vi "Verify as JSON.vi"(7 "Test VI (caller)":string, 8 "error in":errorcluster, 10 "Anything":variant, 11 "TestCase":refnum<class "TestCase.lvclass">) -> (0 "error out":errorcluster, 3 "TestCase":refnum<class "TestCase.lvclass">)   [LabVIEW 2020, in "VITester.Extension.lvlib"]
uses:
  VITester.Extension.lvlib
  <vilib>/addons/_JKI Toolkits/VI Tester/TestCase.llb/TestCase.lvclass
  Approval Tests/Approval Tests.lvlib
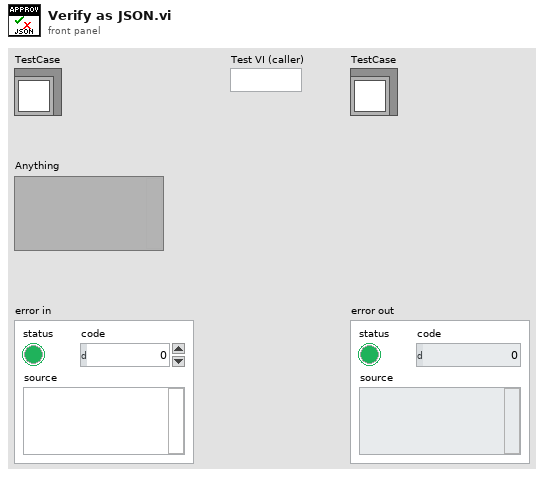
[diagram p1: front panel]
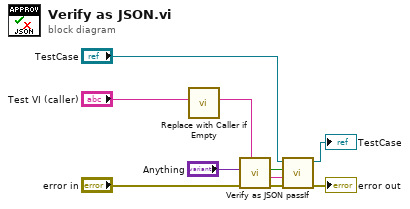
[diagram p0: block diagram]
diagram:
  n1 = call "Replace with Caller if Empty.vi"("Test VI (caller) in"="Test VI (caller)") -> ("Test VI (caller) out"=w2:string)  [unwired: 10 in]
  n2 = call "Verify as JSON.vi"("Test VI (caller)"=w2, "error in"="error in", "Anything"="Anything") -> ("error out"=w9:errorcluster, "Failure Message"=w4:string, "Passed?"=w5:bool)  [unwired: 6 in]
  n3 = call-dynamic "passIf.vi"("error in (no error)"=w9, "message (\"\")"=w4, "pass"=w5, "TestCase in"="TestCase") -> ("error out"=→"error out":errorcluster, "TestCase out"=→"TestCase":refnum<class "TestCase.lvclass">)  [unwired: 6 in]
